vi "Process.vi"(8 "error in":errorcluster, 11 "SMO.SelfTerminating":refnum<class "SMO.SelfTerminatingOverride.lvclass">) -> (0 "error out":errorcluster, 3 "SMO.SelfTerminating out":refnum<class "SMO.SelfTerminatingOverride.lvclass">)   [LabVIEW 2021, in "SMO.SelfTerminatingOverride.lvclass"]
uses:
  SMO.SelfTerminatingOverride.lvclass
  SMO.SelfTerminatingOverride.lvclass/SMO.SelfTerminatingOverride.ctl
  C:/Repositories/SMO/tests/_test-support-SMOs/SMO.SelfTerminating/SMO.SelfTerminating.lvclass
  C:/Repositories/SMO/src/SMO/SMO.lvclass
  C:/Repositories/SMO/tests/_test-support-SMOs/SMO.SelfTerminatingOverride/SMO.SelfTerminatingOverride.lvclass
  src/SMO/Typedefs/Parent Call--Enum.ctl
  src/SMO/SMO.lvclass
  SMO.SelfTerminating/SMO.SelfTerminating.lvclass
panel:
  # "For instructions on how to use the JKI State Machine Objects, examples and video tutorials, visit:\nhttp://jki.net/state-machine-objects/\n\nJKI State Machine Objects™\nhttp://jki.net/state-machine-objects/\nCopyright (C) 2005-2015, JKI <info@jki.net>\nALL RIGHTS RESERVED"
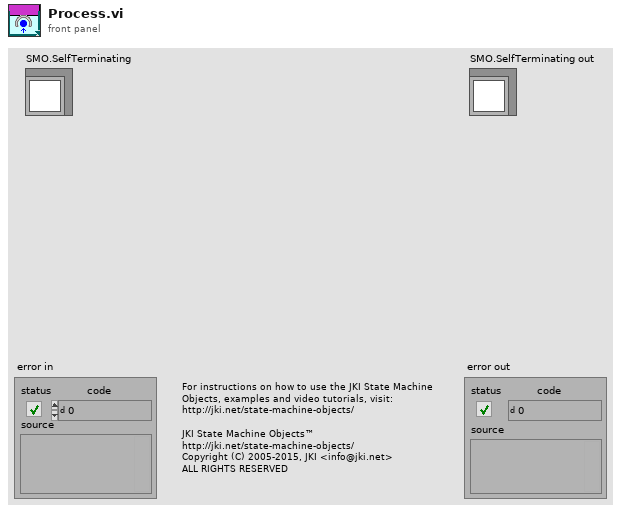
[diagram p1: front panel]
types:
  T1 = typedef "smo.lvlib/SMO.lvclass/Parent Call--Enum.ctl" = enum16{"Allows parent to run", "Does not request parent to run"}
  T2 = typedef "smo.lvlib/SMO.lvclass/Protected Events.ctl" = cluster{"StopProcesses":refnum<user-event>, "AbortProcesses":refnum<user-event>, "Config Changed":refnum<user-event>, "Dependency":refnum<user-event>}
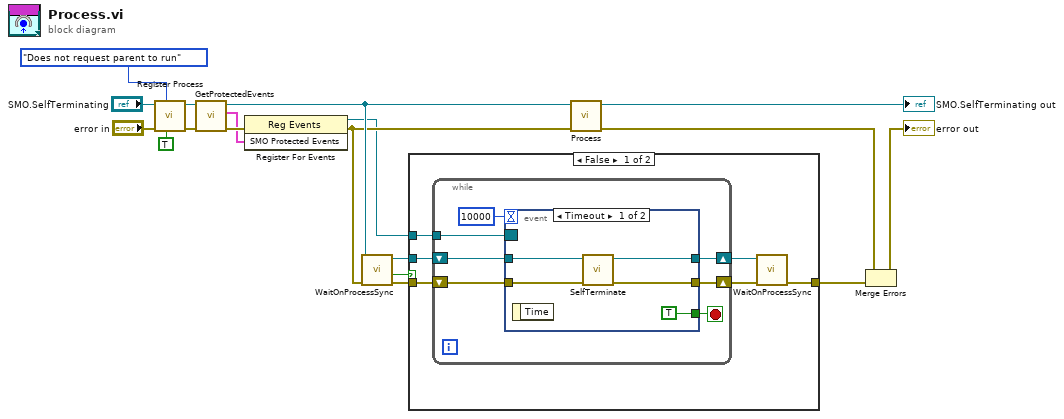
[diagram p0: block diagram]
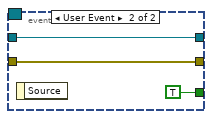
[diagram p2: hidden frame]
diagram:
  n1 = call "Register Process.vi"("Forces Self to Run (F)"=TRUE, "Parent Call"=Parent_Call--Enum."Does not request parent to run", "error in (no error)"="error in", "SMO"="SMO.SelfTerminating") -> ("error out"=w9:errorcluster, "SMO out"=w11:refnum<class "SMO.SelfTerminatingOverride.lvclass">)  [unwired: 6 in]
  n2 = call "GetProtectedEvents.vi"("error in (no error)"=w9, "SMO"=w11) -> ("error out"=w8:errorcluster, "SMO Protected Events"=w6:T2, "SMO out"=w10:refnum<class "SMO.SelfTerminatingOverride.lvclass">)  [unwired: 7 in]
  n3 = register-events(error in=w8, w6) -> (reference out=w5:refnum<event-registration>, error out=w7:errorcluster)  [unwired: 1 in]
  n4 = call "WaitOnProcessSync.vi"("error in (no error)"=w7, "SMO"=w10) -> ("error out"=w3:errorcluster, "Don't run?"=w2:bool, "SMO out"=w4:refnum<class "SMO.SelfTerminatingOverride.lvclass">)  [unwired: 7 in]
  n5 = case shown="False" w2 {
    tunnel: [w24 w40] -> w12
    tunnel: w5 -> [w23 _]
    tunnel: w4 -> [w22 _]
    tunnel: w3 -> [w21 w40]
    frame False {
      n6 = while {
        tunnel: w23 -> [w30]
        shift-right: [w28] -> w20
        shift-left: w22 -> [w29]
        shift-right: [w26] -> w19
        shift-left: w21 -> [w27]
        stop <- w25 stop-if-true
        n7 = event shown="[0] Timeout" {
          selector: w30 -> [_ _]
          dyn-events: _ -> [_ _]
          timeout: 10000 -> [_ _]
          tunnel: w29 -> [w34 w39]
          tunnel: [w33 w39] -> w28
          tunnel: w27 -> [w35 w38]
          tunnel: [w32 w38] -> w26
          tunnel: [TRUE TRUE] -> w25
          event Timeout {
            n8 = event-data() -> ()  [unwired: 1 in, 1 out]
            n9 = call "SelfTerminate.vi"("error in (no error)"=w35, "SMO in"=w34) -> ("error out"=w32:errorcluster, "SMO in"=w33:refnum<class "SMO.SelfTerminatingOverride.lvclass">)  [unwired: 8 in]
          }
          event User Event {
            n10 = event-data() -> ()  [unwired: 1 in, 1 out]
          }
        }
      }
      n11 = call "WaitOnProcessSync.vi"("error in (no error)"=w19, "SMO"=w20) -> ("error out"=w24:errorcluster)  [unwired: 7 in, 2 out]
    }
    frame True {
    }
  }
  n12 = call-parent "Process.vi"("error in"=w7, "SMO.SelfTerminating"=w10) -> ("error out"=w17:errorcluster, "SMO.SelfTerminating out"=→"SMO.SelfTerminating out":refnum<class "SMO.SelfTerminatingOverride.lvclass">)  [unwired: 8 in]
  n13 = Merge Errors(w17, w12) -> (→"error out":errorcluster)
